vi "InstrumentFactory.vi"(6 "InstrumentsToSimulate":string[](array[string]), 8 "error in":errorcluster, 10 "InstrumentConfig(ini)":string, 11 "AllInstrumentDriver":refnum<class "VdInstrument.lvclass">[](array[class])) -> (0 "error out":errorcluster, 2 "InstrumentNamesCreated":string[](array[string]), 3 "InstrumentCreated":refnum<class "VdInstrument.lvclass">[](array[class]))   [LabVIEW 2020, in "VdInstrument.lvclass"]
uses:
  VdInstrument.lvclass
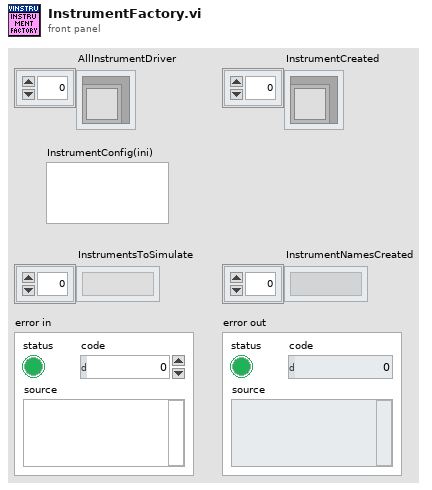
[diagram p1: front panel]
types:
  T1 = typedef "VdInstrument.lvclass/InstrumentType.ctl" = enum16{"NotDefined", "AirflowController", "AnalogInput", "AnalogOutput", "AutoCollimator", "BeamProfiler", "DMM", "DigitalControl", "DigitalInput", "DisplacementSensor", "Encoder", "ForceSensor", "FrequencyCounter", "FunctionGenerator", "GelDispensingRobot", "GlueDispenser", "Hexapod", "IRCamera", "ImageGenerator", "LabelPrinter", "LightController", "LightIndicator", "Load", "Multimeter", "OpticalAttenuatorPowerMeter", "OpticalChannelMonitor", "OpticalLaser", "OpticalPolarizationController", "OpticalPowerAttenuator", "OpticalPowerMeter", "OpticalSpectrumAnalyzer", "PDLMeter", "PolarisationScrambler", "PolarizationAnalyzer", "PositionSensitiveDetector", "PowerSupply", "PressureController", "Robot", "SLRCamera", "ScrewdriverController", "SignalAnalyzer", "SignalGenerator", "SixAxisStage", "SolderingStation", "SpectrumAnalyzer", "StepperMotor", "Stirrer", "SweptWavelengthSystem", "Switch", "TemperatureChamber", "TemperatureController", "TemperatureSensor", "TunableLaser", "UVCuring", "UsbHub", "VisionCamera", "WavelengthMeter", "WeldingLaser"}
  T2 = cluster{"InstrumentType":T1, "DriverName":string}
  T3 = typedef "VdInstrument.lvclass/InstrumentConfig.ctl" = cluster{"InstrumentName":string, "InstrumentType":T1, "DriverName":string, "Adress":string, "Parmameters":string[], "Values":string[]}
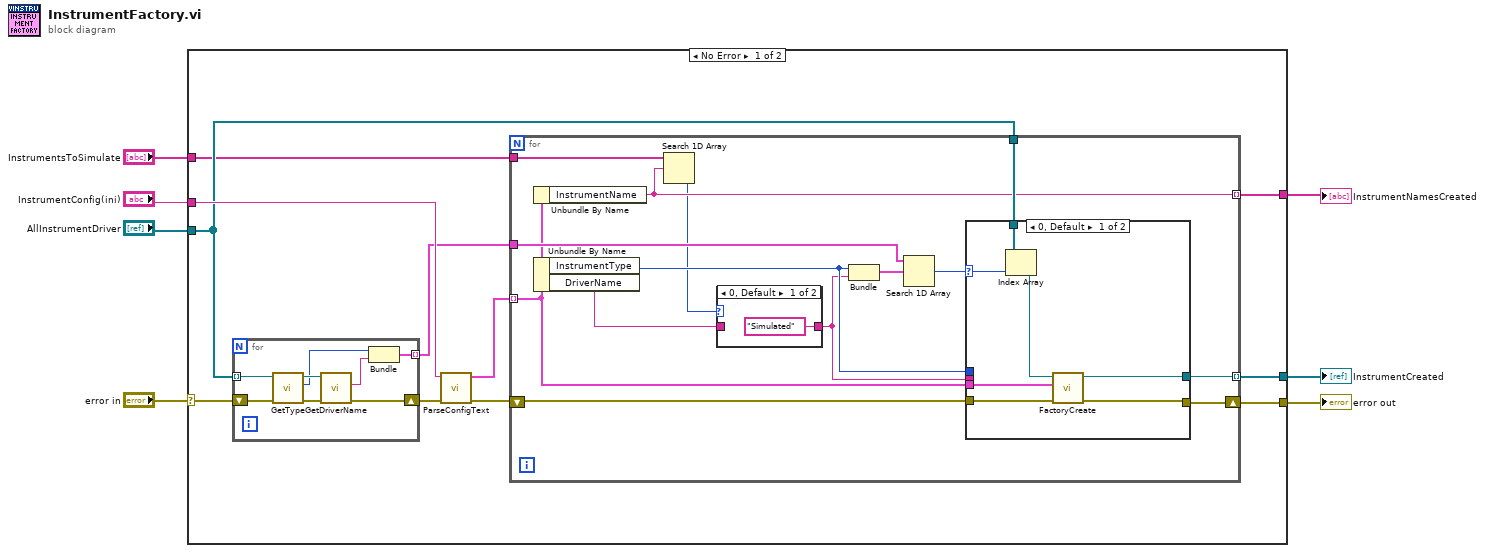
[diagram p0: block diagram]
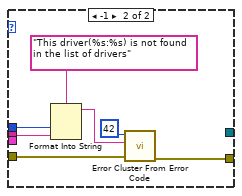
[diagram p3: hidden frame]
diagram:
  n1 = case shown="No Error" "error in" {
    selector: "error in" -> [w18 w57]
    tunnel: [w9 w57] -> w6
    tunnel: "AllInstrumentDriver" -> [w12 _]
    tunnel: "InstrumentConfig(ini)" -> [w17 _]
    tunnel: [w11 _] -> w3
    tunnel: [w10 _] -> w2
    tunnel: "InstrumentsToSimulate" -> [w8 _]
    frame No Error {
      n2 = for {
        tunnel: w12 -> [w26] mode=indexing
        shift-right: [w22] -> w16
        shift-left: w18 -> [w23]
        tunnel: [w19] -> w14 mode=indexing
        n3 = call-dynamic "GetType.vi"("Error In"=w23, "reference in"=w26) -> ("Error Out"=w25:errorcluster, "InstrumentType"=w21:T1, "reference in"=w24:refnum<class "VdInstrument.lvclass">)  [unwired: 7 in]
        n4 = call-dynamic "GetDriverName.vi"("Error In"=w25, "reference in"=w24) -> ("Error Out"=w22:errorcluster, "DriverName"=w20:string)  [unwired: 7 in, 1 out]
        n5 = Bundle("InstrumentType"=w21, "DriverName"=w20) -> (w19:T2)  [unwired: 1 in]
      }
      n6 = call "ParseConfigText.vi"("error in (no error)"=w16, "InstrumentConfig(ini)"=w17) -> ("error out"=w13:errorcluster, "Instruments"=w15:T3[])  [unwired: 8 in]
      n7 = for {
        tunnel: w15 -> [w32] mode=indexing
        tunnel: w14 -> [w39]
        shift-right: [w35] -> w9
        shift-left: w13 -> [w37]
        tunnel: w12 -> [w34]
        tunnel: [w33] -> w11 mode=indexing
        tunnel: [w31] -> w10 mode=indexing
        tunnel: w8 -> [w30]
        n8 = Unbundle By Name(w32) -> ("InstrumentName"=w31:string)
        n9 = Unbundle By Name(w32) -> ("InstrumentType"=w36:T1, "DriverName"=w28:string)
        n10 = Search 1D Array(1D array=w30, element=w31) -> (index of element=w29:i32)  [unwired: 1 in]
        n11 = case shown="0, Default" w29 {
          tunnel: w28 -> [_ w42]
          tunnel: ["Simulated" ("DriverName") w42] -> w27
          frame 0, Default {
          }
          frame -1 {
          }
        }
        n12 = Bundle("InstrumentType"=w36, "DriverName"=w27) -> (w40:T2)  [unwired: 1 in]
        n13 = Search 1D Array(1D array=w39, element=w40) -> (index of element=w38:i32)  [unwired: 1 in]
        n14 = case shown="0, Default" w38 {
          selector: w38 -> [w47 _]
          tunnel: w37 -> [w49 w56]
          tunnel: w36 -> [_ w54]
          tunnel: w27 -> [_ w53]
          tunnel: [w44 w50] -> w35
          tunnel: w34 -> [w48 _]
          tunnel: w32 -> [w45 _]
          tunnel: [w43 _] -> w33
          frame 0, Default {
            n15 = Index Array(array=w48, index=w47) -> (element=w46:refnum<class "VdInstrument.lvclass">)
            n16 = call-dynamic "FactoryCreate.vi"("Error In"=w49, "InstrumentConfig"=w45, "reference in"=w46) -> ("Error Out"=w44:errorcluster, "reference out"=w43:refnum<class "VdInstrument.lvclass">)  [unwired: 7 in]
          }
          frame -1 {
            n17 = Format Into String(format string="This driver(%s:%s) is not found in the list of drivers" ("error message (\"\")"), w54, w53) -> (resulting string=w52:string)  [unwired: 2 in, 1 out]
            n18 = call <vilib>:"Error Cluster From Error Code.vi"("error in (no error)"=w56, "error message (\"\")"=w52, "error code (0)"=42) -> ("error out"=w50:errorcluster)  [unwired: 6 in]
          }
        }
      }
    }
    frame Error {
    }
  }
  "error out" <- w6
  "InstrumentCreated" <- w3
  "InstrumentNamesCreated" <- w2
